vi "TestTarget.vi"(6 "Wiring Spec":T1, 8 "error in (no error)":errorcluster, 10 "Do VI":refnum<vi>, 11 "CS++Actor in":refnum<class "CS++Actor.lvclass">) -> (0 "error out":errorcluster, 3 "CS++Actor out":refnum<class "CS++Actor.lvclass">)   [LabVIEW 2015, in "TestVIs.lvlib"]
uses:
  TestVIs.lvlib
  CSPP_Actor/CS++Actor.lvclass
  CSPP_Actor/CS++Actor.lvclass/CS++Actor.ctl
  <vilib>/Utility/traverseref.llb/TRef TravTarget.ctl
  <vilib>/Utility/traverseref.llb/VI Scripting - Traverse.lvlib
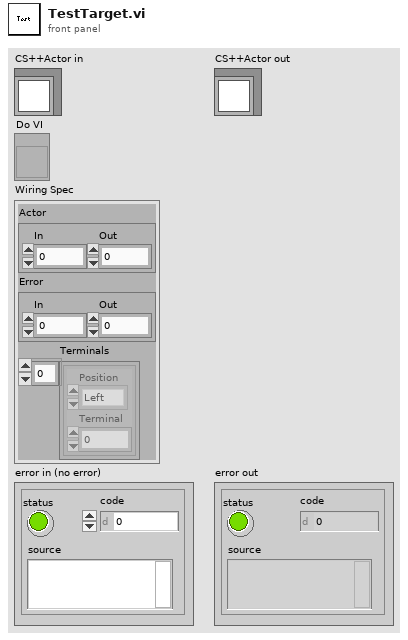
[diagram p1: front panel]
types:
  T1 = cluster{"Actor":cluster{"In":i32, "Out":i32}, "Error":cluster{"In":i32, "Out":i32}, "Terminals":cluster{"Position":enum16{"Left", "Top", "Bottom", "Right"}, "Terminal":i32}[]}
  T2 = enum16{"Replace Class Controls/Constants", "Prepare SubVI", "Wire Method Inputs"}
  T3 = typedef "TRef TravTarget.ctl" = enum16{"FP", "BD", "Other"}
  T4 = cluster{"Position":enum16{"Left", "Top", "Bottom", "Right"}, "Terminal":i32}[]
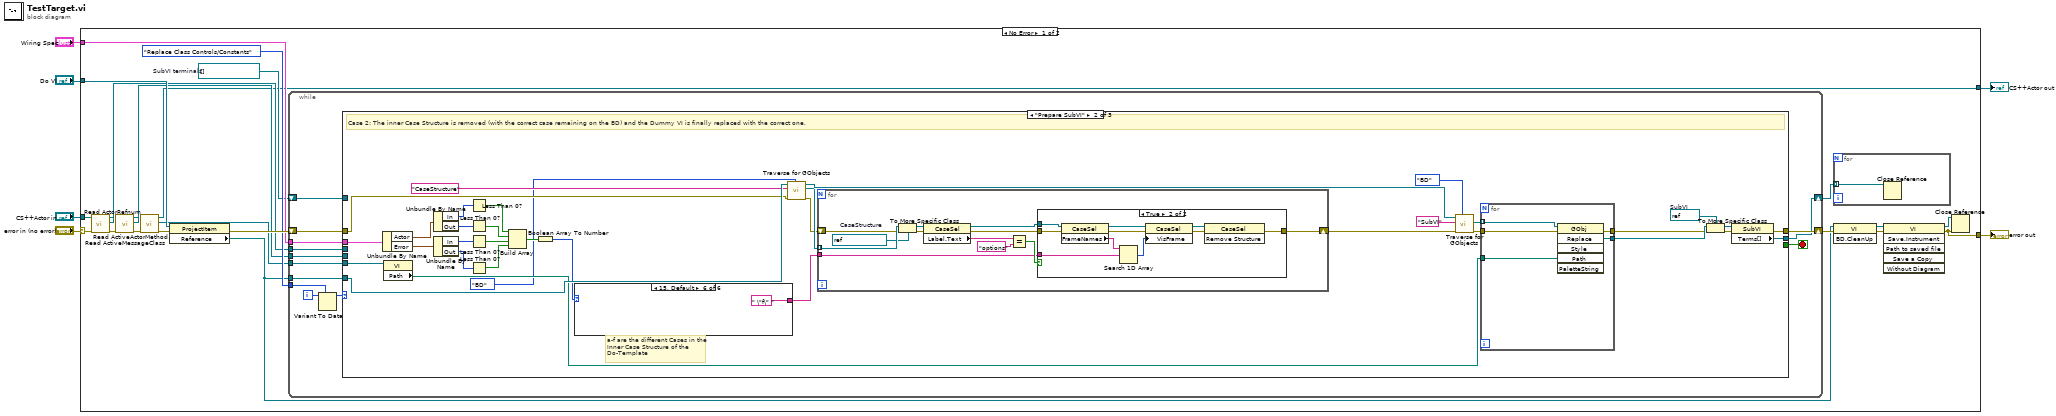
[diagram p0: block diagram]
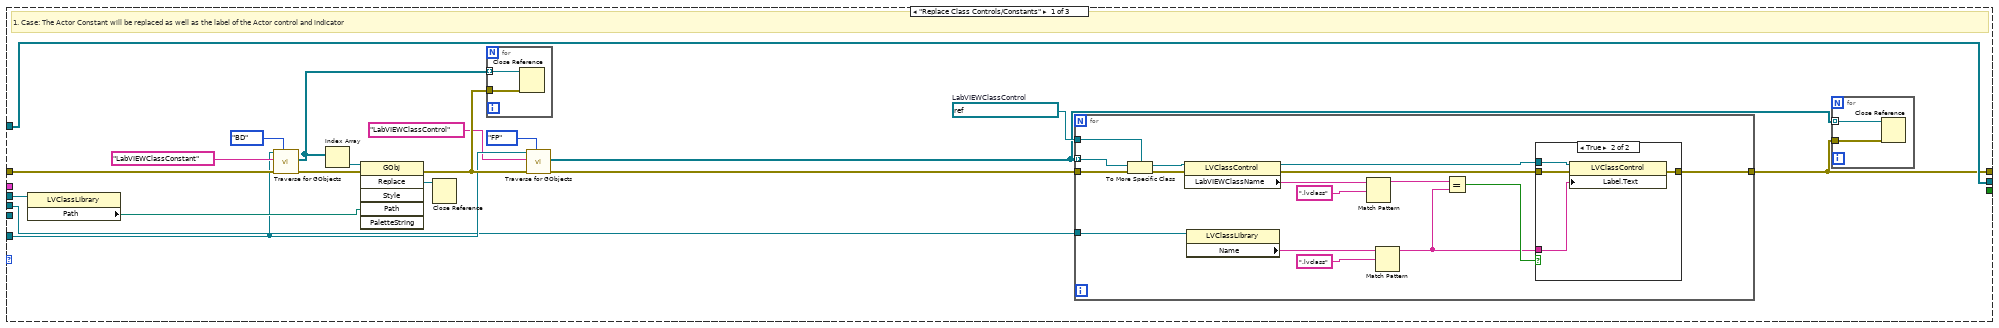
[diagram p2: hidden frame]
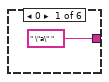
[diagram p5: hidden frame]
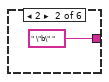
[diagram p6: hidden frame]
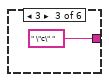
[diagram p7: hidden frame]
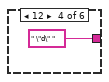
[diagram p8: hidden frame]
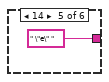
[diagram p9: hidden frame]
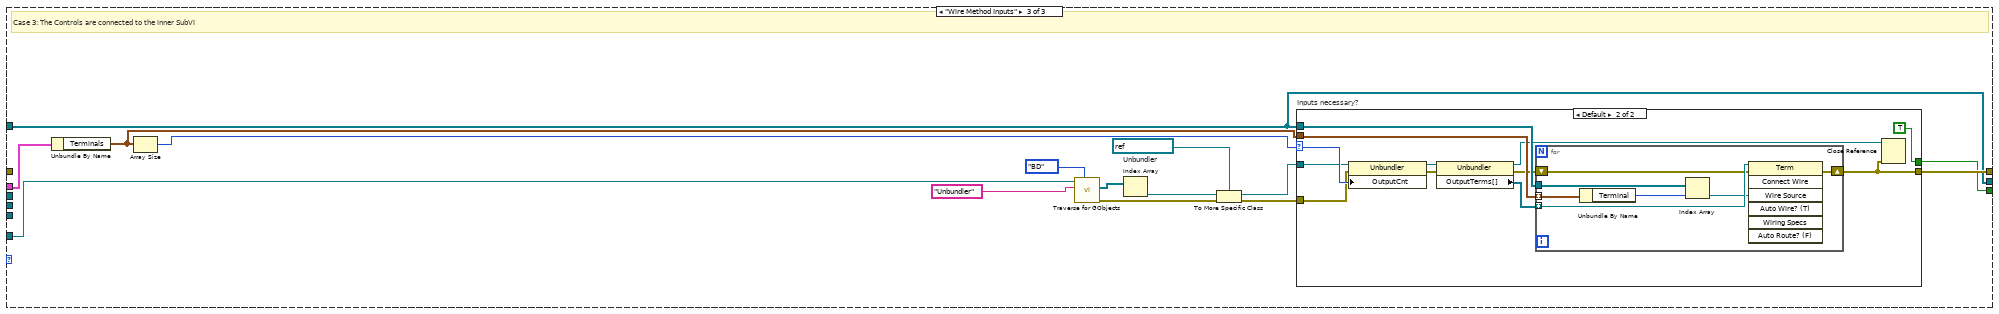
[diagram p10: hidden frame]
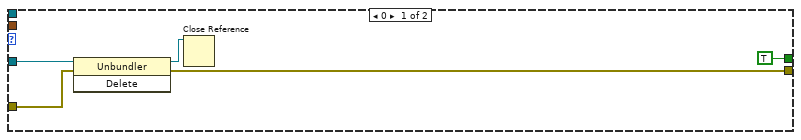
[diagram p11: hidden frame]
diagram:
  n1 = case shown="No Error" "error in (no error)" {
    selector: "error in (no error)" -> [w11 w196]
    tunnel: "Do VI" -> [w29 _]
    tunnel: "Wiring Spec" -> [w27 _]
    tunnel: [w7 w196] -> w4
    tunnel: "CS++Actor in" -> [w21 w197]
    tunnel: [w12 w197] -> w2
    frame No Error {
      w24 = refnum<vi>[] []  # SubVI terminals
      n2 = call "Read ActorRefnum.vi"("error in (no error)"=w11, "CS++Actor in"=w21) -> ("error out"=w18:errorcluster, "ActorRefnum"=w20:refnum<vi>, "CS++Actor out"=w19:refnum<class "CS++Actor.lvclass">)  [unwired: 7 in]
      n3 = call "Read ActiveMessageClass.vi"("error in (no error)"=w18, "CS++Actor in"=w19) -> ("error out"=w15:errorcluster, "ActiveMessageClass"=w17:refnum<vi>, "CS++Actor out"=w16:refnum<class "CS++Actor.lvclass">)  [unwired: 7 in]
      n4 = call "Read ActiveActorMethod.vi"("error in (no error)"=w15, "CS++Actor in"=w16) -> ("error out"=w13:errorcluster, "ActiveActorMethod"=w14:refnum<vi>, "CS++Actor out"=w12:refnum<class "CS++Actor.lvclass">)  [unwired: 7 in]
      n5 = property class="ProjectItem"(reference=w29, error in=w13) -> (error out=w28:errorcluster, "Reference"=w22:refnum<vi>)  [unwired: 1 out]
      n6 = while {
        tunnel: w22 -> [w43]
        tunnel: w27 -> [w41]
        shift-right: [w40] -> w26
        shift-left: w28 -> [w42]
        tunnel: T2."Replace Class Controls/Constants" -> [w38]
        tunnel: w20 -> [w36]
        tunnel: w14 -> [w35]
        shift-right: [w33] -> w23
        shift-left: w24 -> [w32]
        tunnel: w17 -> [w31]
        i -> [w39]
        stop <- w34 stop-if-true
        n7 = Variant To Data(type=w38, Variant=w39) -> (data=w37:T2)  [unwired: 1 in, 1 out]
        n8 = case shown="\"Prepare SubVI\"" w37 {
          tunnel: w43 -> [w51 w122 w171]
          tunnel: w42 -> [w56 w121 _]
          tunnel: w41 -> [_ w120 w164]
          tunnel: [w44 w88 w160] -> w40
          tunnel: w36 -> [w57 _ _]
          tunnel: w35 -> [_ w119 _]
          tunnel: [_ _ w157] -> w34
          tunnel: [w53 w118 w159] -> w33
          tunnel: w32 -> [w53 _ w159]
          tunnel: w31 -> [w46 _ _]
          frame "Replace Class Controls/Constants" {
            w49 = refnum<vi> refnum  # LabVIEWClassControl
            # "1. Case: The Actor Constant will be replaced as well as the label of the Actor control and indicator"
            n9 = property class="LVClassLibrary"(reference=w57) -> ("Path"=w60:path)  [unwired: 1 in, 2 out]
            n10 = call <vilib>:"Traverse for GObjects.vi"("Traverse Target"=TRef_TravTarget."BD", "error in (no error)"=w56, "Class Name"="LabVIEWClassConstant", "VI Refnum"=w51) -> ("error out"=w61:errorcluster, "References"=w55:refnum<vi>[])  [unwired: 4 in, 2 out]
            n11 = Index Array(array=w55) -> (element=w59:refnum<vi>)  [unwired: 1 in]
            n12 = invoke class="GObj" method="Replace"(reference=w59, error in=w61, "Path"=w60) -> (error out=w52:errorcluster, "Replace"=w54:refnum<vi>)  [unwired: 3 in, 4 out]
            n13 = Close Reference(reference=w54) -> ()  [unwired: 1 in, 1 out]
            n14 = for {
              tunnel: w55 -> [w66] mode=indexing
              tunnel: w52 -> [w65]
              n15 = Close Reference(reference=w66, error in (no error)=w65) -> ()  [unwired: 1 out]
            }
            n16 = call <vilib>:"Traverse for GObjects.vi"("Traverse Target"=TRef_TravTarget."FP", "error in (no error)"=w52, "Class Name"="LabVIEWClassControl", "VI Refnum"=w51) -> ("error out"=w47:errorcluster, "References"=w45:refnum<vi>[])  [unwired: 4 in, 2 out]
            n17 = for {
              tunnel: w49 -> [w82]
              tunnel: w47 -> [w81]
              tunnel: w45 -> [w80] mode=indexing
              tunnel: w46 -> [w75]
              tunnel: [w77] -> w44
              n18 = To More Specific Class(target class=w82, reference=w80, error in=w81) -> (specific class reference=w76:refnum<vi>, error out=w78:errorcluster)
              n19 = property class="LVClassControl"(reference=w76, error in=w78) -> (reference out=w79:refnum<vi>, error out=w67:errorcluster, "LabVIEWClassName"=w69:string)
              n20 = property class="LVClassLibrary"(reference=w75) -> ("Name"=w73:string)  [unwired: 1 in, 2 out]
              n21 = Match Pattern(string=w69, regular expression=".lvclass") -> (before substring=w68:string)  [unwired: 1 in, 3 out]
              n22 = Match Pattern(string=w73, regular expression=".lvclass") -> (before substring=w72:string)  [unwired: 1 in, 3 out]
              n23 = Equal?(x=w68, y=w72) -> (x = y?=w74:bool)
              n24 = case shown="True" w74 {
                tunnel: w79 -> [_ w87]
                tunnel: [w83 w84] -> w77
                tunnel: w72 -> [_ w86]
                tunnel: w67 -> [w83 w85]
                frame False {
                }
                frame True {
                  n25 = property class="LVClassControl"(reference=w87, error in=w85, "Label.Text"=w86) -> (error out=w84:errorcluster)  [unwired: 1 out]
                }
              }
            }
            n26 = for {
              tunnel: w45 -> [w64] mode=indexing
              tunnel: w44 -> [w63]
              n27 = Close Reference(reference=w64, error in (no error)=w63) -> ()  [unwired: 1 out]
            }
          }
          frame "Prepare SubVI" {
            w91 = refnum<vi> refnum  # SubVI
            # "a-f are the different Cases in the\nInner Case Structure of the \nDo-Template"
            # "Case 2: The inner Case Structure is removed (with the correct case remaining on the BD) and the Dummy VI is finally replaced with the correct one."
            n28 = Unbundle By Name(w120) -> ("Actor"=w113:cluster{"In":i32, "Out":i32}, "Error"=w112:cluster{"In":i32, "Out":i32})
            n29 = property class="VI"(reference=w119) -> ("Path"=w114:path)  [unwired: 1 in, 2 out]
            n30 = Unbundle By Name(w113) -> ("In"=w111:i32, "Out"=w110:i32)
            n31 = Unbundle By Name(w112) -> ("In"=w109:i32, "Out"=w108:i32)
            n32 = Less Than 0?(x=w111) -> (x < 0?=w107:bool)
            n33 = Less Than 0?(x=w110) -> (x < 0?=w106:bool)
            n34 = Less Than 0?(x=w109) -> (x < 0?=w105:bool)
            n35 = Less Than 0?(x=w108) -> (x < 0?=w104:bool)
            n36 = Build Array(w107, w106, w105, w104) -> (w103:bool[])
            n37 = Boolean Array To Number(Boolean array=w103) -> (number=w102:u32)
            n38 = case shown="15, Default" w102 {
              tunnel: [" \"a\" " " \"b\" " " \"c\" " " \"d\" " " \"e\" " " \"f\" "] -> w97
              frame 0 {
              }
              frame 2 {
              }
              frame 3 {
              }
              frame 12 {
              }
              frame 14 {
              }
              frame 15, Default {
              }
            }
            n39 = call <vilib>:"Traverse for GObjects.vi"("Traverse Target"=TRef_TravTarget."BD", "error in (no error)"=w121, "Class Name"="CaseStructure", "VI Refnum"=w122) -> ("error out"=w96:errorcluster, "References"=w98:refnum<vi>[], "dup VI Refnum"=w101:refnum<vi>)  [unwired: 4 in, 1 out]
            n40 = for {
              tunnel: w98 -> [w134] mode=indexing
              tunnel: w97 -> [w125]
              shift-right: [w123] -> w95
              shift-left: w96 -> [w124]
              w133 = refnum<vi> refnum  # CaseStructure
              n41 = To More Specific Class(target class=w133, reference=w134, error in=w124) -> (specific class reference=w132:refnum<vi>, error out=w131:errorcluster)
              n42 = property class="CaseSel"(reference=w132, error in=w131) -> (reference out=w127:refnum<vi>, error out=w126:errorcluster, "Label.Text"=w130:string)
              n43 = Equal?(x=w130, y="options") -> (x = y?=w128:bool)
              n44 = case shown="True" w128 {
                tunnel: w127 -> [_ w143]
                tunnel: w126 -> [w135 w141]
                tunnel: w125 -> [_ w137]
                tunnel: [w135 w136] -> w123
                frame False {
                }
                frame True {
                  n45 = property class="CaseSel"(reference=w143, error in=w141) -> (reference out=w142:refnum<vi>, error out=w140:errorcluster, "FrameNames"=w139:string[])
                  n46 = Search 1D Array(1D array=w139, element=w137) -> (index of element=w138:i32)  [unwired: 1 in]
                  n47 = property class="CaseSel"(reference=w142, error in=w140, "VisFrame"=w138) -> (reference out=w145:refnum<vi>, error out=w144:errorcluster)
                  n48 = invoke class="CaseSel" method="Remove Structure"(reference=w145, error in=w144) -> (error out=w136:errorcluster)  [unwired: 1 in, 2 out]
                }
              }
            }
            n49 = call <vilib>:"Traverse for GObjects.vi"("Traverse Target"=TRef_TravTarget."BD", "error in (no error)"=w95, "Class Name"="SubVI", "VI Refnum"=w101) -> ("error out"=w90:errorcluster, "References"=w115:refnum<vi>[])  [unwired: 4 in, 2 out]
            n50 = for {
              tunnel: w115 -> [w156] mode=indexing
              tunnel: w114 -> [w155]
              tunnel: [w154] -> w93
              tunnel: w90 -> [w153]
              tunnel: [w152] -> w89
              n51 = invoke class="GObj" method="Replace"(reference=w156, error in=w153, "Path"=w155) -> (error out=w152:errorcluster, "Replace"=w154:refnum<vi>)  [unwired: 3 in, 4 out]
            }
            n52 = To More Specific Class(target class=w91, reference=w93, error in=w89) -> (specific class reference=w94:refnum<vi>, error out=w92:errorcluster)
            n53 = property class="SubVI"(reference=w94, error in=w92) -> (error out=w88:errorcluster, "Terms[]"=w118:refnum<vi>[])  [unwired: 1 out]
          }
          frame "Wire Method Inputs" {
            w165 = refnum<vi> refnum  # Unbundler
            # "Case 3: The Controls are connected to the inner SubVI"
            n54 = Unbundle By Name(w164) -> ("Terminals"=w158:T4)
            n55 = Array Size(array=w158) -> (size(s)=w163:i32)
            n56 = call <vilib>:"Traverse for GObjects.vi"("Traverse Target"=TRef_TravTarget."BD", "Class Name"="Unbundler", "VI Refnum"=w171) -> ("error out"=w166:errorcluster, "References"=w168:refnum<vi>[])  [unwired: 5 in, 2 out]
            n57 = Index Array(array=w168) -> (element=w167:refnum<vi>)  [unwired: 1 in]
            n58 = To More Specific Class(target class=w165, reference=w167, error in=w166) -> (specific class reference=w162:refnum<vi>, error out=w161:errorcluster)
            n59 = case "Inputs necessary?" shown="Default" w163 {
              selector: w163 -> [_ w183]
              tunnel: w162 -> [w176 w181]
              tunnel: w159 -> [_ w186]
              tunnel: w161 -> [w175 w178]
              tunnel: [w174 w179] -> w160
              tunnel: w158 -> [_ w188]
              tunnel: [TRUE TRUE] -> w157
              frame 0 {
                n60 = invoke class="Unbundler" method="Delete"(reference=w176, error in=w175) -> (reference out=w173:refnum<vi>, error out=w174:errorcluster)  [unwired: 1 in, 1 out]
                n61 = Close Reference(reference=w173) -> ()  [unwired: 1 in, 1 out]
              }
              frame Default {
                n62 = property class="Unbundler"(reference=w181, error in=w178, "OutputCnt"=w183) -> (reference out=w184:refnum<vi>, error out=w182:errorcluster)
                n63 = property class="Unbundler"(reference=w184, error in=w182) -> (reference out=w180:refnum<vi>, error out=w185:errorcluster, "OutputTerms[]"=w187:refnum<vi>[])
                n64 = for {
                  tunnel: w188 -> [w190] mode=indexing
                  tunnel: w187 -> [w195] mode=indexing
                  tunnel: w186 -> [w194]
                  shift-right: [w191] -> w179
                  shift-left: w185 -> [w192]
                  n65 = Unbundle By Name(w190) -> ("Terminal"=w189:i32)
                  n66 = Index Array(array=w194, index=w189) -> (element=w193:refnum<vi>)
                  n67 = invoke class="Term" method="Connect Wire"(reference=w195, error in=w192, "Wire Source"=w193) -> (error out=w191:errorcluster)  [unwired: 4 in, 6 out]
                }
                n68 = Close Reference(reference=w180, error in (no error)=w179) -> ()  [unwired: 1 out]
              }
            }
          }
        }
      }
      n69 = for {
        tunnel: w23 -> [w30] mode=indexing
        n70 = Close Reference(reference=w30) -> ()  [unwired: 1 in, 1 out]
      }
      n71 = invoke class="VI" method="BD.CleanUp"(reference=w22, error in=w26) -> (reference out=w10:refnum<vi>, error out=w8:errorcluster)  [unwired: 1 in, 1 out]
      n72 = invoke class="VI" method="Save.Instrument"(reference=w10, error in=w8) -> (reference out=w9:refnum<vi>, error out=w7:errorcluster)  [unwired: 4 in, 4 out]
      n73 = Close Reference(reference=w9, error in (no error)=w7) -> ()  [unwired: 1 out]
    }
    frame Error {
    }
  }
  "error out" <- w4
  "CS++Actor out" <- w2
